vi "LVDimInterface.error_message.vi"(0 "type of dialog (no dialog: 0)":u16(ring) items=["no dialog", "OK message", "continue or stop message"], 2 "add message to source":bool, 5 "error in (no error)":errorcluster) -> (14 "message":string="No Error", 15 "code out":i32, 16 "error?":bool, 19 "error out":errorcluster)   [LabVIEW 2015, in "LVDimInterface.lvlib"]
doc: "Contains all the instrument-specific error codes and descriptions.\n\nIn case of an error, this VI adds the error message to the error source.\nOptionaly, an error message pops up.\n\nHistory: 15-FEB-2006, Dietrich Beck\n\nCopyright (C)\nGesellschaft für Schwerionenforschung, GSI\nPlanckstr. 1\n64291 Darmstadt\nGermany\n\nContact: D.Beck@gsi.de \n\nThis program is free software; you can redistribute it and/or modify it under the terms of the \nGNU General Public License as published by the Free Software Foundation; either version 2 of the license, or (at your option) any later version.\n\nThis program is distributed in the hope that it will be useful, but WITHOUT ANY WARRANTY; without even the implied warranty of MERCHANTABILITY or FITNESS FOR A PARTICULAR PURPOSE. See the GNU General License for more details (http://www.gnu.org).\n\nGesellschaft für Schwerionenforschung, GSI\nPlanckstr. 1, 64291 Darmstadt, Germany\nFor all questions and ideas contact: D. Beck, M.Richter@gsi.de or H.Brand@gsi.de.\nLast update: 05-APR-2004"
uses:
  LVDimInterface.lvlib
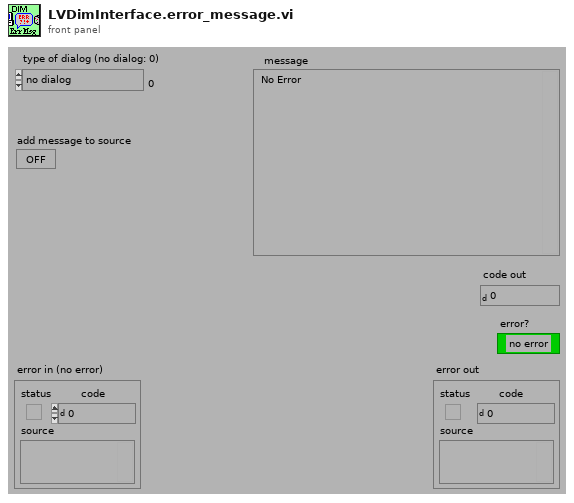
[diagram p1: front panel]
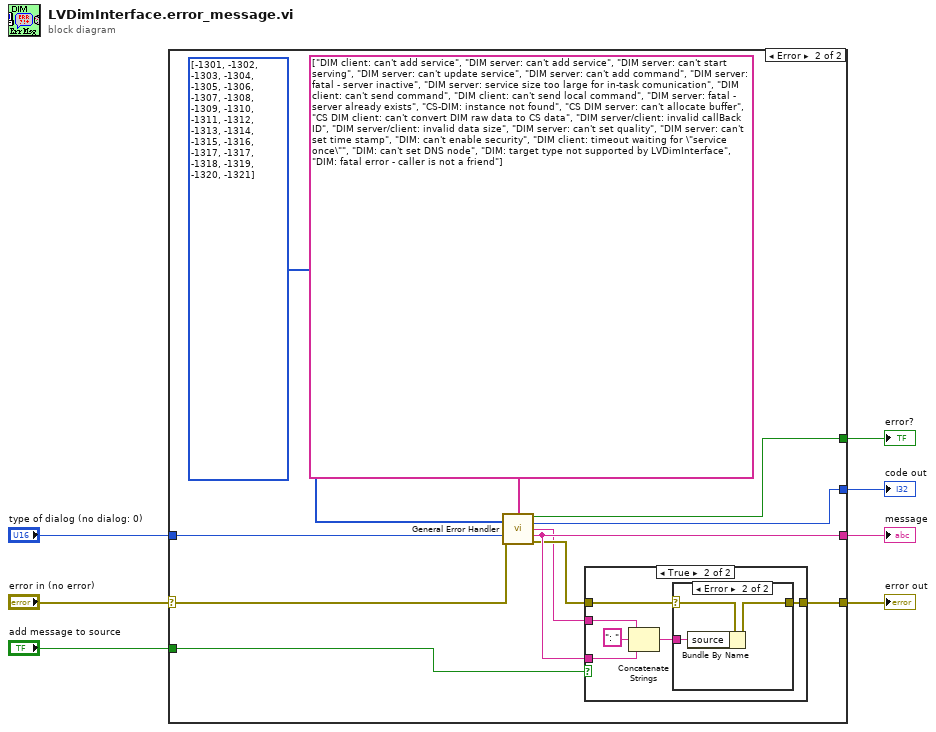
[diagram p0: block diagram]
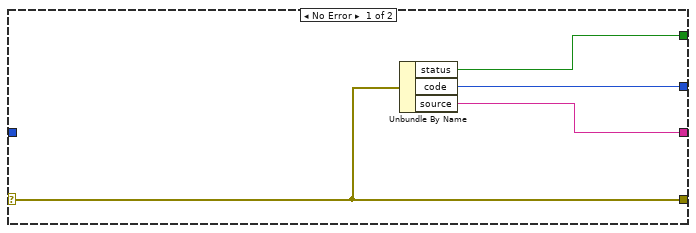
[diagram p2: hidden frame]
diagram:
  n1 = case shown="Error" "error in (no error)" {
    selector: "error in (no error)" -> [w11 w12]
    tunnel: [w11 w22] -> w7
    tunnel: "type of dialog (no dialog: 0)" -> [_ w21]
    tunnel: [w8 w20] -> w5
    tunnel: [w9 w19] -> w4
    tunnel: [w10 w18] -> w3
    tunnel: "add message to source" -> [_ w13]
    frame No Error {
      n2 = Unbundle By Name(w11) -> ("status"=w10:bool, "code"=w9:i32, "source"=w8:string)
    }
    frame Error {
      n3 = call <vilib>:"General Error Handler.vi"("[user-defined codes]"=i32[] [-1301, -1302, -1303, -1304, -1305, -1306, -1307, -1308, -1309, -1310, -1311, -1312, -1313, -1314, -1315, -1316, -1317, -1317, -1318, -1319, -1320, -1321], "[user-defined descriptions]"=string[] ["DIM client: can't add service", "DIM server: can't add service", "DIM server: can't start serving", "DIM server: can't update service", "DIM server: can't add command", "DIM server: fatal - server inactive", "DIM server: service size too large for in-task comunication", "DIM client: can't send command", "DIM client: can't send local command", "DIM server: fatal - server already exists", "CS-DIM: instance not found", "CS DIM server: can't allocate buffer", "CS DIM client: can't convert DIM raw data to CS data", "DIM server/client: invalid callBack ID", "DIM server/client: invalid data size", "DIM server: can't set quality", "DIM server: can't set time stamp", "DIM: can't enable security", "DIM client: timeout waiting for \"service once\"", "DIM: can't set DNS node", "DIM: target type not supported by LVDimInterface", "DIM: fatal error - caller is not a friend"], "type of dialog (OK msg:1)"=w21, "error in (no error)"=w12) -> ("error?"=w18:bool, "code out"=w19:i32, "source out"=w14:string, "message"=w20:string, "error out"=w15:errorcluster)  [unwired: 7 in]
      n4 = case shown="True" w13 {
        tunnel: [w23 w29] -> w22
        tunnel: w20 -> [_ w24]
        tunnel: w15 -> [w23 w25]
        tunnel: w14 -> [_ w28]
        frame False {
        }
        frame True {
          n5 = Concatenate Strings(w28, ": " ("Substring"), w24) -> (w26:string)
          n6 = case shown="Error" w25 {
            selector: w25 -> [w30 w31]
            tunnel: [w30 w33] -> w29
            tunnel: w26 -> [_ w32]
            frame No Error {
            }
            frame Error {
              n7 = Bundle By Name(cluster=w31, "source"=w32) -> (w33:errorcluster)
            }
          }
        }
      }
    }
  }
  "error out" <- w7
  "message" <- w5
  "code out" <- w4
  "error?" <- w3
